vi "Measurement Logic.vi"() -> ()   [LabVIEW 2021, in "Linearity_DAC.lvlib"]
uses:
  Linearity_DAC.lvlib
  Measurement Configuration.ctl
  Measurement Results.ctl
  <vilib>/MeasurementLink/MeasurementLink Measurement Server/Measure Call Context/Measure Call Context.lvclass
  <instrlib>/niDMM/nidmm.llb/niDMM Configure Measurement Digits.vi
panel:
  out "measure call context out":refnum<class "Measure Call Context.lvclass">
  in  "measure call context in":refnum<class "Measure Call Context.lvclass">
  out "measurement results":T1
  in  "measurement configuration":T2={"Digital resource"="", "Sweep start code"=32, "Sweep stop code"=3968, "DAC channel"=0, "Full scale range"=5, "DMM resource"="", "DMM resolution"=5.5, "DMM range"=10.0}
  out "error out":errorcluster
  in  "error in":errorcluster
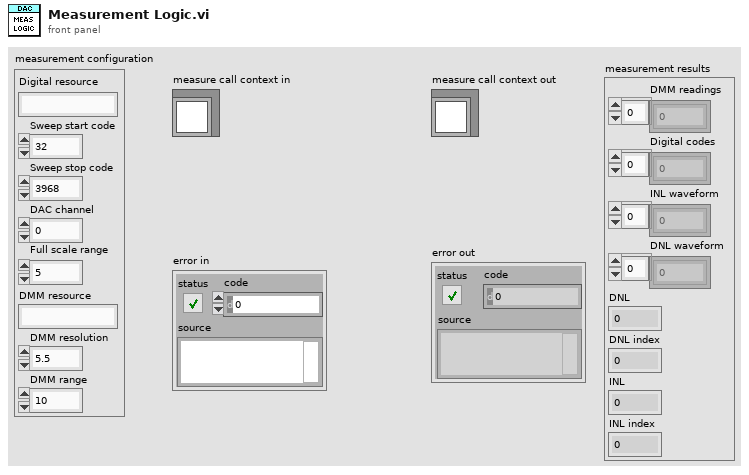
[diagram p1: front panel]
types:
  T1 = typedef "Linearity_DAC.lvlib/Measurement Results.ctl" = cluster{"DMM readings":dbl[], "Digital codes":u32[], "INL waveform":dbl[], "DNL waveform":dbl[], "DNL":dbl, "DNL index":u32, "INL":dbl, "INL index":u32}
  T2 = typedef "Linearity_DAC.lvlib/Measurement Configuration.ctl" = cluster{"Digital resource":string, "Sweep start code":u32, "Sweep stop code":u32, "DAC channel":u32, "Full scale range":u32, "DMM resource":string, "DMM resolution":dbl, "DMM range":dbl}
  T3 = cluster{"Number of commands":u16, "Digital commands":i16[], "Command size":u16, "Sweep start code":u32}
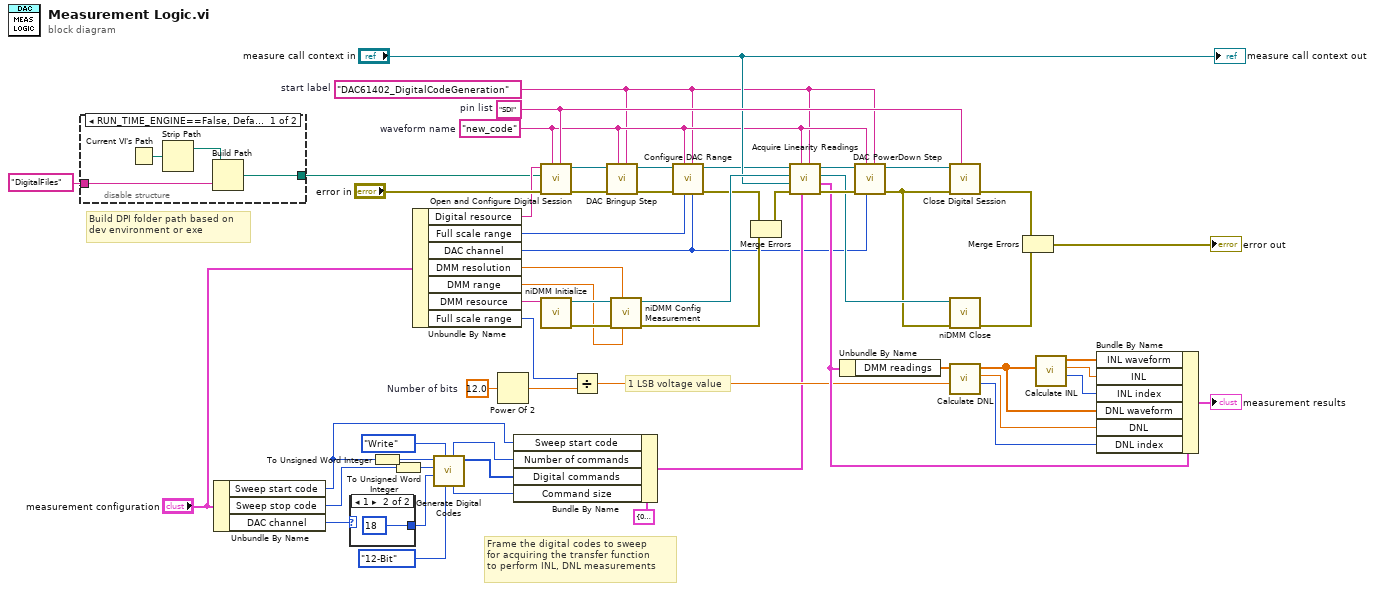
[diagram p0: block diagram]
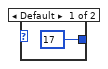
[diagram p2: hidden frame]
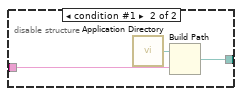
[diagram p3: hidden frame]
diagram:
  w26 = 12.0  # Number of bits
  w4 = "DAC61402_DigitalCodeGeneration"  # start label
  w44 = "SDI"  # pin list
  w5 = "new_code"  # waveform name
  # "Frame the digital codes to sweep\nfor acquiring the transfer function\nto perform INL, DNL measurements"
  # "1 LSB voltage value"
  # "Build DPI folder path based on\ndev environment or exe"
  n1 = disable-structure shown="RUN_TIME_ENGINE==False, Default" {
    disable-tunnel: "DigitalFiles" -> [w61 w65]
    disable-tunnel: [w60 w64] -> w27
    frame condition #0 (active) {
      n2 = Current VI's Path() -> (path=w63:path)
      n3 = Strip Path(path=w63) -> (stripped path=w62:path)  [unwired: 1 out]
      n4 = Build Path(base path=w62, name or relative path=w61) -> (appended path=w60:path)
    }
    frame condition #1 {
      n5 = call <vilib>:"Application Directory.vi"() -> ("Application Directory"=w66:path)
      n6 = Build Path(base path=w66, name or relative path=w65) -> (appended path=w64:path)
    }
  }
  n7 = Unbundle By Name("measurement configuration") -> ("Sweep start code"=w11:u32, "Sweep stop code"=w20:u32, "DAC channel"=w19:u32)
  n8 = case shown="1" w19 {
    tunnel: [u8 17 u8 18] -> w21
    frame Default {
    }
    frame 1 {
    }
  }
  n9 = To Unsigned Word Integer(number=w11) -> (unsigned 16bit integer=w18:u16)
  n10 = To Unsigned Word Integer(number=w20) -> (unsigned 16bit integer=w17:u16)
  n11 = Unbundle By Name("measurement configuration") -> ("Digital resource"=w58:string, "Full scale range"=w2:u32, "DAC channel"=w3:u32, "DMM resolution"=w52:dbl, "DMM range"=w51:dbl, "DMM resource"=w55:string, "Full scale range"=w1:u32)
  n12 = call "Generate Digital Codes.vi"("Input Code Bit"=enum16{"16-Bit", "12-Bit"}."12-Bit", "Command"=enum16{"Read", "Write"}."Write", "Address"=w21, "End code"=w17, "Start code"=w18) -> ("Digital commands"=w14:i16[], "Command size"=w13:u16, "Number of commands"=w12:u16)  [unwired: 4 in]
  n13 = Power Of 2(x=w26) -> (2^x=w25:dbl)
  n14 = Bundle By Name(cluster=T3 {"Number of commands"=0, "Digital commands"=[], "Command size"=0, "Sweep start code"=0} ("Digital command info"), "Sweep start code"=w11, "Number of commands"=w12, "Digital commands"=w14, "Command size"=w13) -> (w10:T3)
  n15 = call "Open and Configure Digital Session.vi"("pin list"=w44, "waveform name"=w5, "error in"="error in", "Digital pattern folder"=w27, "Digital resource"=w58) -> ("error out"=w56:errorcluster, "Digital session"=w57:refnum<k15>)  [unwired: 5 in]
  n16 = call <instrlib>:"niDMM Initialize.vi"("Instrument Descriptor"=w55) -> ("error out"=w53:errorcluster, "instrument handle out"=w54:refnum<k15>)  [unwired: 9 in]
  n17 = Divide(x=w1, y=w25) -> (x/y=w24:dbl)
  n18 = call "DAC Bringup Step.vi"("start label"=w4, "waveform name"=w5, "error in"=w56, "Digital session"=w57) -> ("error out"=w7:errorcluster, "Digital session out"=w9:refnum<k15>)  [unwired: 6 in]
  n19 = call-poly <instrlib>:"niDMM Config Measurement.vi"("Range"=w51, "Resolution in Digits"=w52, "error in (no error)"=w53, "instrument handle"=w54) -> ("error out"=w30:errorcluster, "instrument handle out"=w50:refnum<k15>)  [unwired: 6 in]
  n20 = call "Configure DAC Range.vi"("DAC Channel"=w3, "start label"=w4, "Full scale range"=w2, "waveform name"=w5, "error in"=w7, "Digital session"=w9) -> ("error out"=w6:errorcluster, "Digital session out"=w8:refnum<k15>)  [unwired: 4 in]
  n21 = Merge Errors(w6, w30) -> (w29:errorcluster)
  n22 = call "Acquire Linearity Readings.vi"("start label"=w4, "Digital command info"=w10, "waveform name"=w5, "error in"=w29, "measure call context in"="measure call context in", "DMM session"=w50, "Digital session"=w8) -> ("error out"=w48:errorcluster, "measurement results"=w42:T1, "DMM session out"=w47:refnum<k15>, "Digital session out"=w49:refnum<k15>)  [unwired: 1 in]
  n23 = Unbundle By Name(w42) -> ("DMM readings"=w43:dbl[])
  n24 = call "DAC PowerDown Step.vi"("start label"=w4, "DAC channel"=w3, "waveform name"=w5, "error in"=w48, "Digital sesssion"=w49) -> ("error out"=w45:errorcluster, "Digital session out"=w46:refnum<k15>)  [unwired: 5 in]
  n25 = call "Close Digital Session.vi"("pin list"=w44, "error in"=w45, "Digital session"=w46) -> ("error out"=w33:errorcluster)  [unwired: 8 in]
  n26 = call <instrlib>:"niDMM Close.vi"("error in (no error)"=w45, "instrument handle"=w47) -> ("error out"=w34:errorcluster)  [unwired: 9 in]
  n27 = call "Calculate DNL.vi"("1 Ideal LSB value"=w24, "DAC Analog readings"=w43) -> ("DNL index"=w39:i32, "DNL"=w40:dbl, "DNL waveform"=w41:dbl[])  [unwired: 7 in]
  n28 = Merge Errors(w33, w34) -> (→"error out":errorcluster)
  n29 = call "Calculate INL.vi"("DNL"=w41) -> ("Max INL"=w38:i32, "INL"=w37:dbl, "INL waveform"=w36:dbl[])  [unwired: 8 in]
  n30 = Bundle By Name(cluster=w42, "INL waveform"=w36, "INL"=w37, "INL index"=w38, "DNL waveform"=w41, "DNL"=w40, "DNL index"=w39) -> (→"measurement results":T1)
  "measure call context out" <- "measure call context in"
